vi "Get Global MetaData Channels Section.vi"(8 "error in (no error)":errorcluster, 11 "Item Ref in":T1 format="%.0x") -> (0 "error out":errorcluster, 2 "Item Ref":T1 format="%.0x", 3 "Item Ref out":T1 format="%.0x")   [LabVIEW 2019, in "Instrument Addon System Explorer.lvlib"]
uses:
  Instrument Addon System Explorer.lvlib
  <vilib>/NI VeriStand/Custom Device Tools/Custom Device Utility Library/Custom Device Utility Library.lvlib
  <vilib>/NI VeriStand/Custom Device Tools/Custom Device Utility Library/NI VeriStand - Search for Item by GUID.vi
  Addon Shared/Constants.vi
  Addon Shared/Instrument Addon Shared.lvlib
  <vilib>/NI VeriStand/Custom Device API/Custom Device API.lvlib
  <vilib>/NI VeriStand/Custom Device API/Custom Device Item Ref.ctl
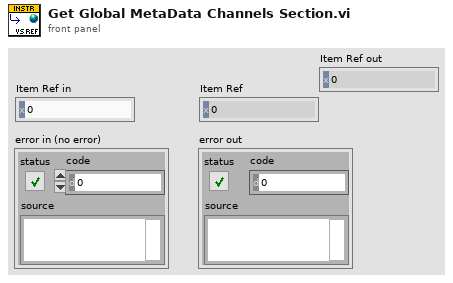
[diagram p1: front panel]
types:
  T1 = typedef "Custom Device API.lvlib/Custom Device Item Ref.ctl" = u64
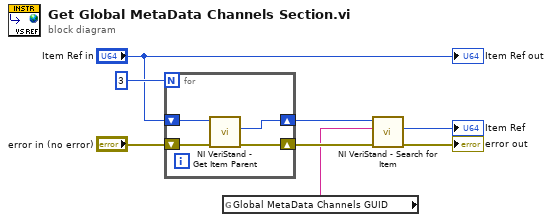
[diagram p0: block diagram]
diagram:
  n1 = for {
    N: 3 -> [_]
    shift-right: [w10] -> w6
    shift-left: "Item Ref in" -> [w12]
    shift-right: [w9] -> w5
    shift-left: "error in (no error)" -> [w11]
    n2 = call <vilib>:"NI VeriStand - Get Item Parent.vi"("error in (no error)"=w11, "Item Ref in"=w12) -> ("error out"=w9:errorcluster, "Parent Ref"=w10:T1)  [unwired: 6 in, 2 out]
  }
  n3 = global read "Constants.vi" "Global MetaData Channels GUID"() -> (w1:string)
  n4 = call-poly <vilib>:"NI VeriStand - Search for Item.vi"("error in"=w5, "Item GUID"=w1, "Section Ref in"=w6) -> ("error out"=→"error out":errorcluster, "Item Ref"=→"Item Ref":T1)  [unwired: 5 in, 2 out]
  "Item Ref out" <- "Item Ref in"
